vi "FPGAController_v3.vi"() -> ()   [LabVIEW 2013]
uses:
  <vilib>/rvi/interface/nirviOpenFPGA/nirviOpenFPGA.xnode
  <vilib>/rvi/interface/nirviMethod/nirviMethod.xnode
  <vilib>/rvi/interface/nirviReadWriteControl/nirviReadWriteControl.xnode
  <vilib>/rvi/interface/nirviCloseFPGA/nirviCloseFPGA.xnode
  ver1(FPGA)_7_8_2013.vi
  <vilib>/addons/database/NI_Database_API.lvlib
  <vilib>/addons/database/Recordset.llb/Rec Fetch Recordset Data (R).vi
  <vilib>/addons/database/Connection.llb/Conn Execute.vi
  <vilib>/addons/database/_DB Variant To Data/Database Variant To Data.xnode
  <vilib>/addons/database/Recordset.llb/Rec Destroy - Connection.vi
  <vilib>/Utility/miscctls.llb/LVPointTypeDef.ctl
  FPGA Bitfiles/correlationwithf_FPGATarget_ver1(FPGA)214201_RJg2enFNf9w.lvbitx
  <userlib>/_OpenG.lib/comparison/comparison.llb/Boolean Changed__ogtk.vi
  <vilib>/rvi/errors/niLvFpgaMergeErrorWithErrorCode.vi
panel:
  out "Rearm Trigger":bool
  in  "Rearm Trigger":bool
  in  "One Shot Mode":bool
  out "Last Update:":timestamp
  out "Updating FPGA":bool
  out "Sensitivity":dbl
  out "error out":errorcluster
  out "Low Mass Limit":fxp<+,31,17>
  out "High Mass Limit":fxp<+,31,17>
  out "stopping":bool
  in  "Auto Threshold":bool
  out "Peletron (MV)":dbl=2.0
  out "High Mass (kg)":dbl=inf
  out "Low Mass (kg)":dbl
  out "High Charge Limit":i16
  out "Low Charge Limit":i16
  out "High velocity count":i32=210
  out "Low velocity count":i32=21000
  in  "stop":bool
  in  "Peak-Threshold Factor":dbl=3.0
  out "Low Charge Limit (fC)":dbl
  out "High Charge Limit (fC)":dbl=100.0
  out "High Velocity":dbl=100000.0
  out "Low Velocity":dbl=1000.0
  out "Filter 7 Peak":i32=7483
  out "Filter 6 Peak":i32=9863
  out "Filter 5 Peak":i32=13910
  out "Filter 4 Peak":i32=18191
  out "Filter 3 Peak":i32=46254
  out "Filter 2 Peak":i32=120664
  out "Filter 1 Peak":i32=295996
  in  "Filter7 Threshold":i32=-21165
  in  "Filter6 Threshold":i32=-29358
  in  "Filter5 Threshold":i32=-41730
  in  "Filter4 Threshold":i32=-54306
  in  "Filter3 Threshold":i32=-138762
  in  "Filter2 Threshold":i32=-361992
  in  "Filter1 Threshold":i32=-887988
  in  "Zero Peak Values":bool
  in  "Assign Threshold":bool
  in  "Run Mode":bool
  # "Settings"
  # "Dubugging"
  # "Independent Variable"
  # "Low Vel."
  # "High Vel."
  # "Low Q (fC)"
  # "High Q (fC)"
  # "Plate Control While Loop Counter"
  # "Low Mass (kg)"
  # "High Mass (kg)"
  # "Sens. (V/pC)"
  # "Peletron (MV)"
  # "Current Value of Running Average"
  # "Peak Threshold Factor"
  # "Peak Values"
  # "Peak 1"
  # "Peak 2"
  # "Peak 3"
  # "Peak 4"
  # "Peak 5"
  # "Peak 6"
  # "Peak 7"
  # "Thresholds"
  # "Threshold 1"
  # "Threshold 2"
  # "Threshold 3"
  # "Threshold 4"
  # "Threshold 5"
  # "Threshold 6"
  # "Threshold 7"
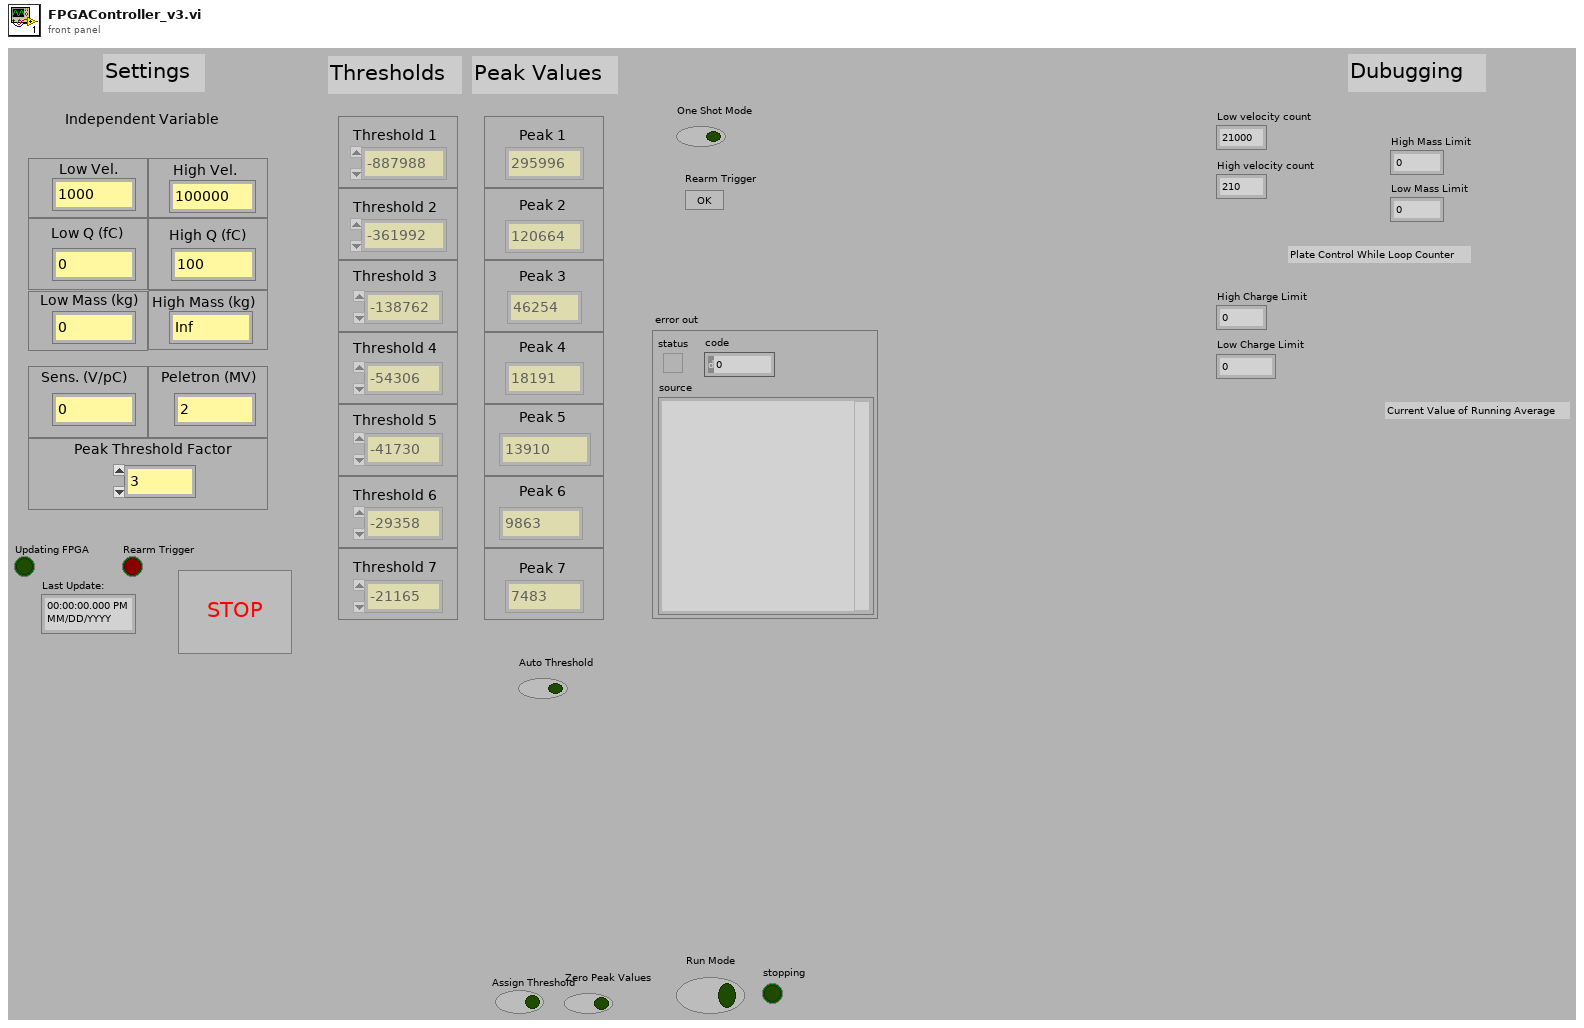
[diagram p1: front panel]
types:
  T1 = typedef "LVPointTypeDef.ctl" = cluster{"Horizontal":i16, "Vertical":i16}
  T2 = enum8{"Enabled", "Disabled", "Disabled and Grayed Out"}
  T3 = typedef "NI_Database_API.lvlib/Conn ObjectReference.ctl" = refnum<k1>
  T4 = cluster{"Filter 1 Peak":i32, "Filter 2 Peak":i32, "Filter 3 Peak":i32, "Filter 4 Peak":i32, "Filter 5 Peak":i32, "Filter 6 Peak":i32, "Filter 7 Peak":i32}
  T5 = typedef "NI_Database_API.lvlib/Rec ObjectReference.ctl" = refnum<k1>
  T6 = cluster{"Numeric":dbl, "Numeric":dbl, "Numeric":dbl, "Numeric":dbl, "Numeric":dbl, "Numeric":dbl, dbl, dbl, "Value":dbl}
  T7 = cluster{"Low Velocity Count":i32, "High Velocity Count":i32, "Low Charge Limit (ADC ticks)":i16, "High Charge Limit (ADC ticks)":i16, "Low Mass (ADC*cycle^2)":i64, "High Mass (ADC*cycle^2)":i64, "Mult":fxp<+,16,7>, "Mult Use?":bool}
  T8 = cluster{"Filter 1 Detector 3 Correlation":void, "Filter 2 Detector 3 Correlation":void, "Filter 3 Detector 3 Correlation":void, "Filter 4 Detector 3 Correlation":void, "Filter 5 Detector 3 Correlation":void, "Filter 6 Detector 3 Correlation":void, "Filter 7 Detector 3 Correlation":void}
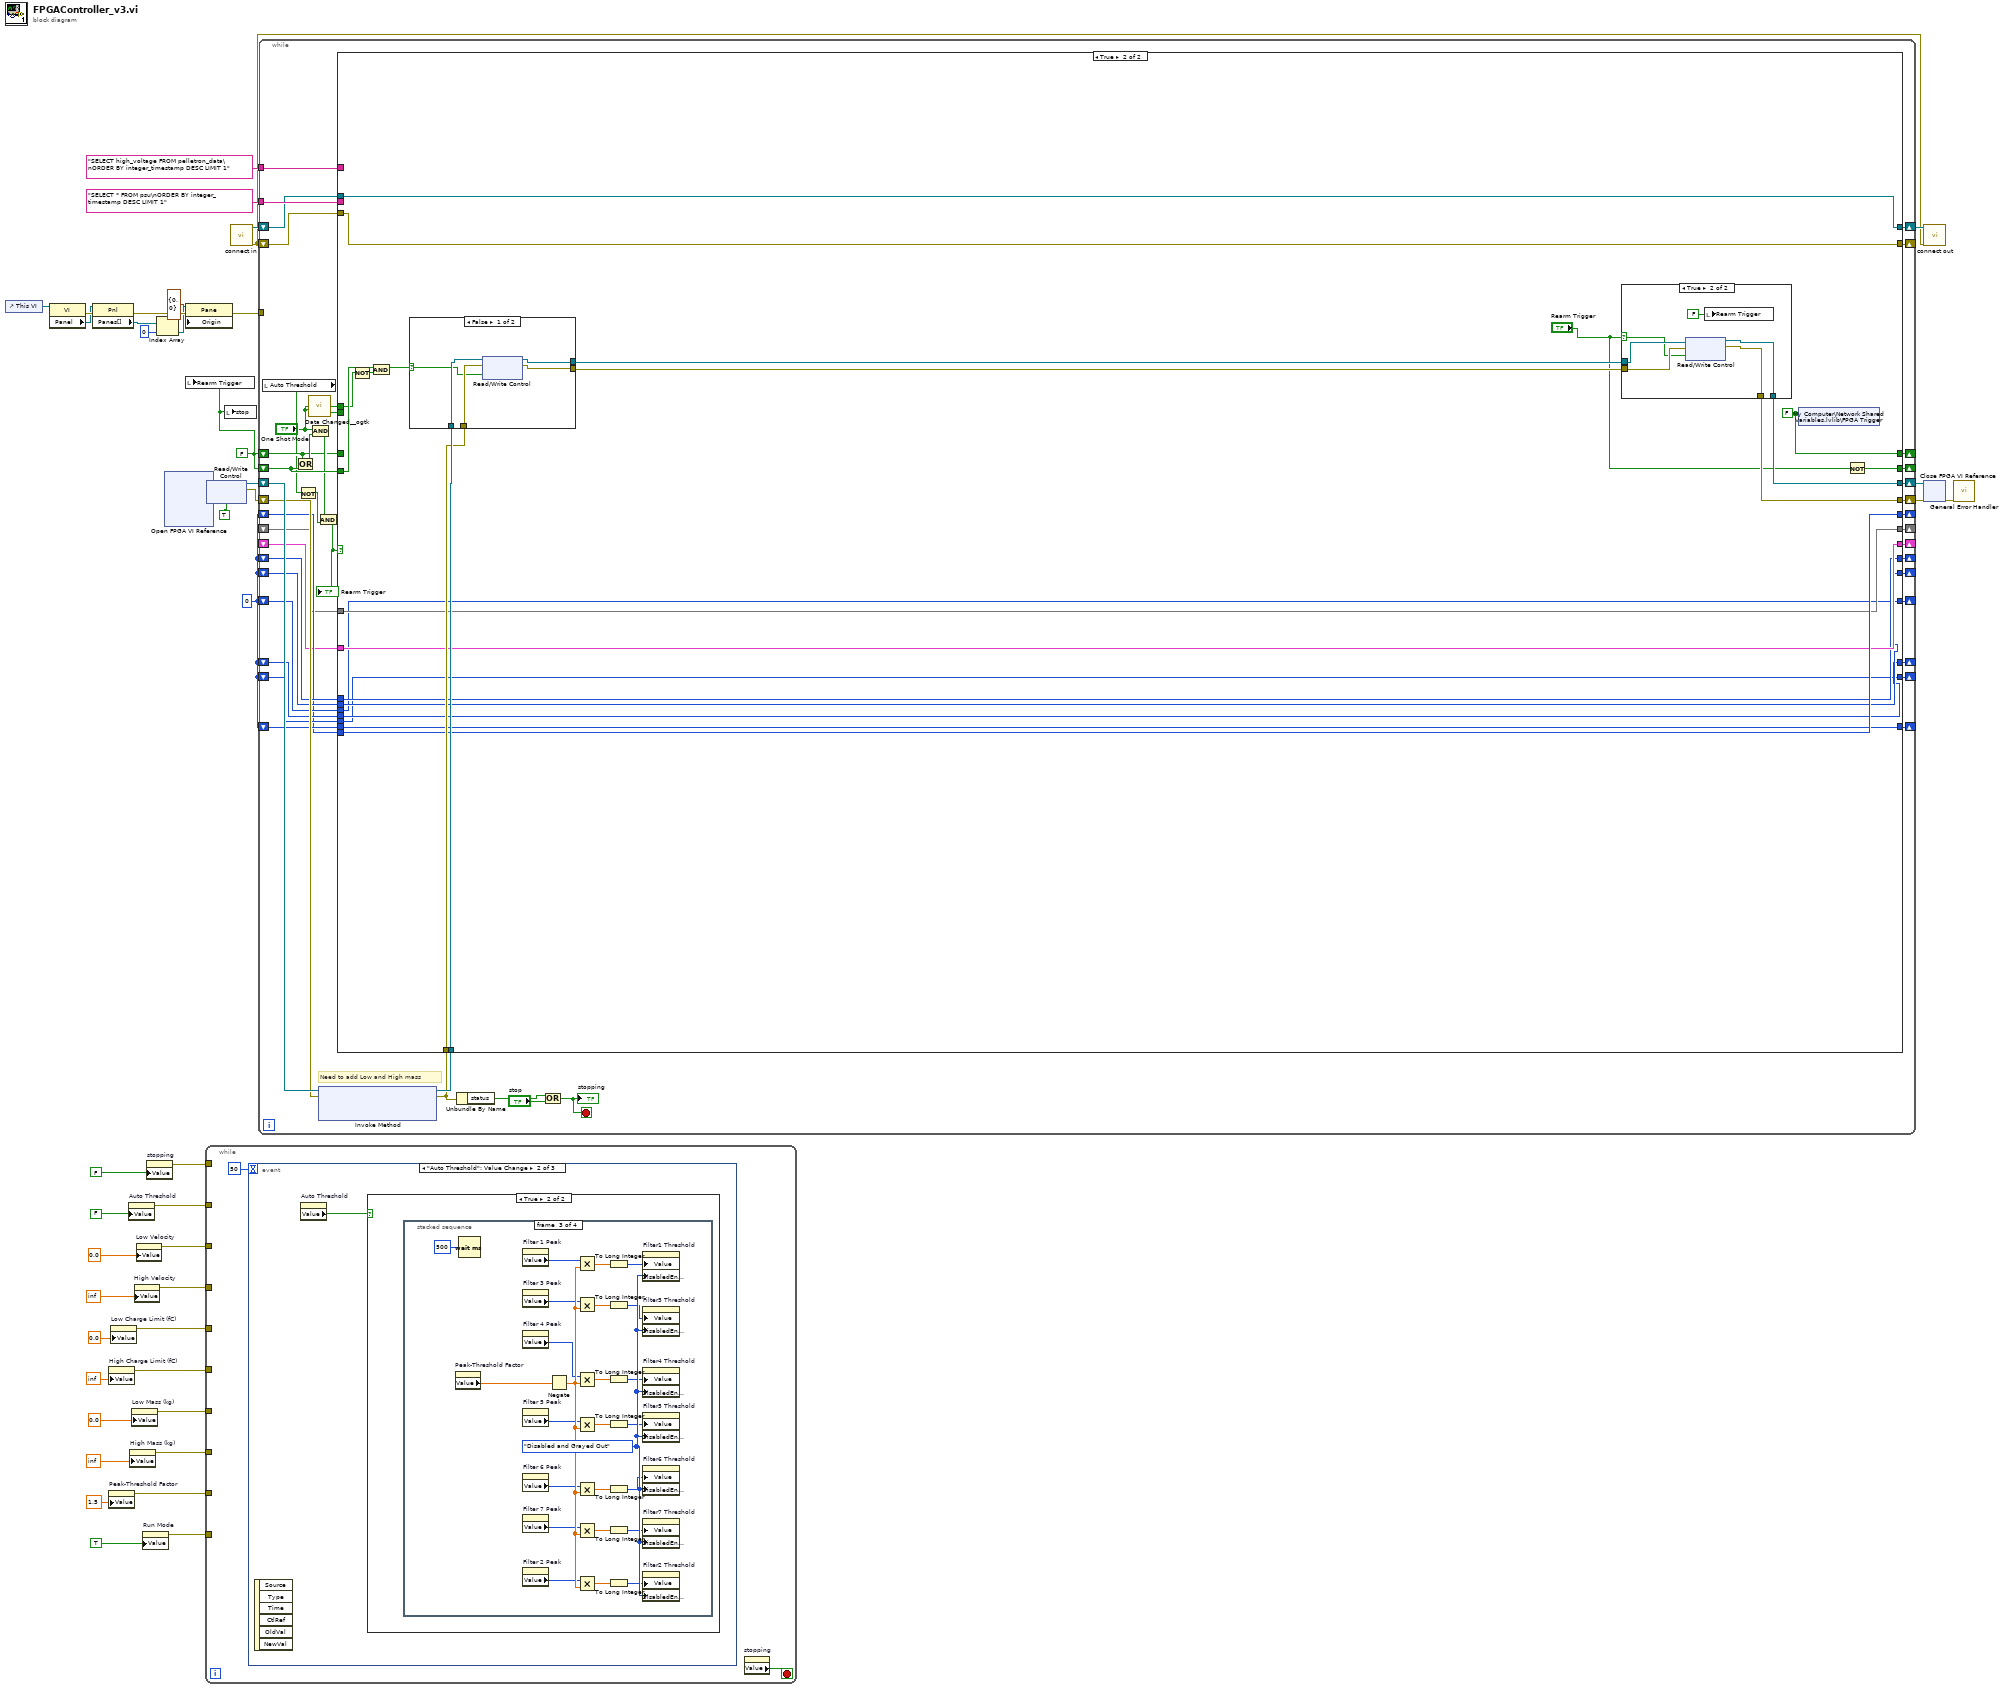
[diagram p0: block diagram]
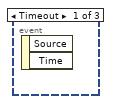
[diagram p2: hidden frame]
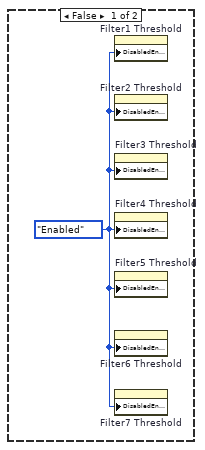
[diagram p3: hidden frame]
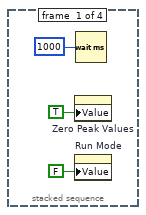
[diagram p4: hidden frame]
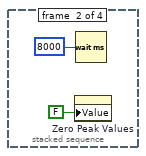
[diagram p5: hidden frame]
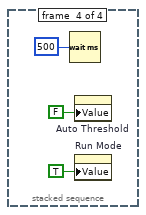
[diagram p6: hidden frame]
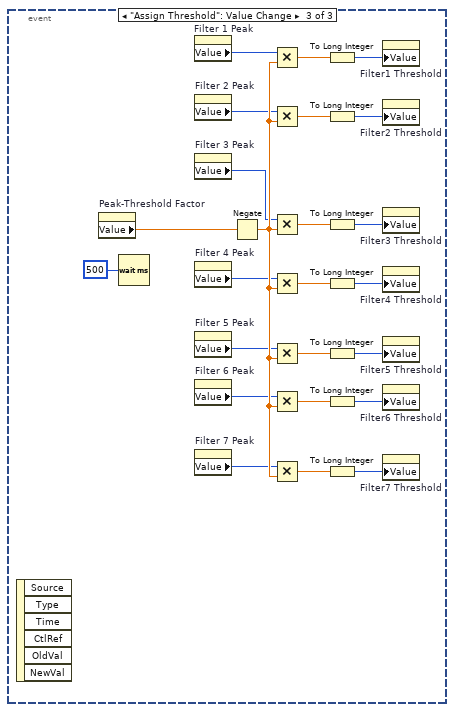
[diagram p7: hidden frame]
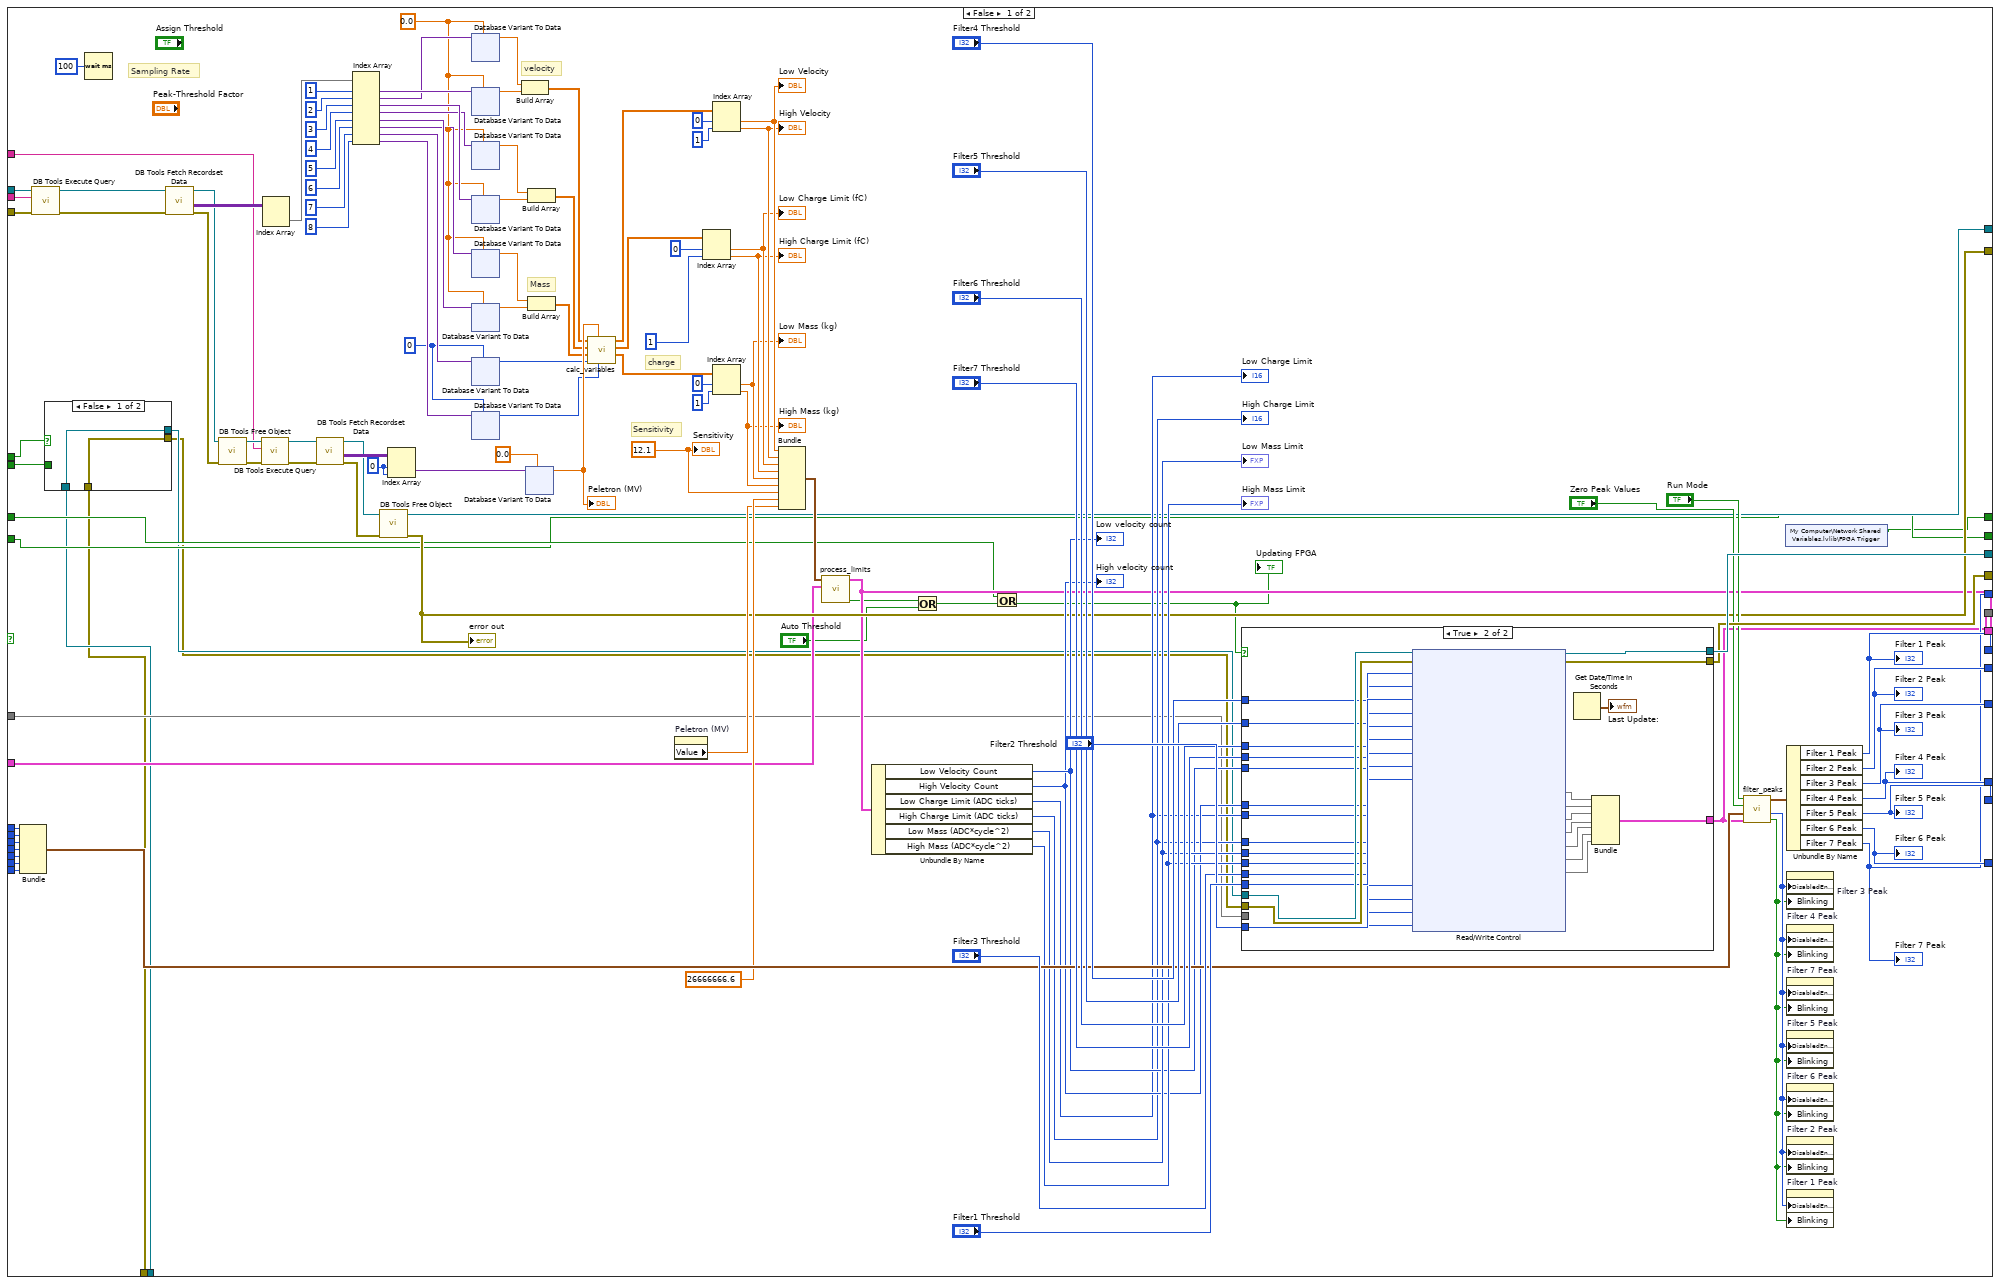
[diagram p8: hidden frame]
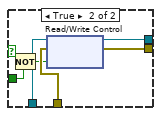
[diagram p9: hidden frame]
diagram:
  w6 = FALSE
  w43 = 0
  n1 = control-ref of="This VI"() -> (w15:refnum<vi>)
  n2 = property class="VI"(reference=w15) -> (error out=w14:errorcluster, "Panel"=w13:refnum<vi>)  [unwired: 1 in, 1 out]
  n3 = property class="Pnl"(reference=w13, error in=w14) -> (error out=w12:errorcluster, "Panes[]"=w11:refnum<vi>[])  [unwired: 1 out]
  n4 = property on="High Charge Limit (fC)" class="DigNum (strict)"("Value"=inf ("High Charge Limit (fC)")) -> (error out=w30:errorcluster)  [unwired: 2 in, 1 out]
  n5 = property on="Peak-Threshold Factor" class="DigNum (strict)"("Value"=1.5 ("Peak-Threshold Factor")) -> (error out=w24:errorcluster)  [unwired: 2 in, 1 out]
  n6 = property on="Low Charge Limit (fC)" class="DigNum (strict)"("Value"=0.0 ("Low Charge Limit (fC)")) -> (error out=w32:errorcluster)  [unwired: 2 in, 1 out]
  n7 = property on="Auto Threshold" class="Bool (strict)"("Value"=FALSE ("Auto Threshold")) -> (error out=w38:errorcluster)  [unwired: 2 in, 1 out]
  n8 = property on="High Mass (kg)" class="DigNum (strict)"("Value"=inf ("High Mass (kg)")) -> (error out=w26:errorcluster)  [unwired: 2 in, 1 out]
  n9 = property on="Low Mass (kg)" class="DigNum (strict)"("Value"=0.0 ("Low Mass (kg)")) -> (error out=w28:errorcluster)  [unwired: 2 in, 1 out]
  n10 = property on="High Velocity" class="DigNum (strict)"("Value"=inf ("High Velocity")) -> (error out=w34:errorcluster)  [unwired: 2 in, 1 out]
  n11 = property on="Low Velocity" class="DigNum (strict)"("Value"=0.0 ("Low Velocity")) -> (error out=w36:errorcluster)  [unwired: 2 in, 1 out]
  n12 = property on="Run Mode" class="Bool (strict)"("Value"=TRUE ("Run Mode")) -> (error out=w22:errorcluster)  [unwired: 2 in, 1 out]
  n13 = property on="stopping" class="Bool (strict)"("Value"=FALSE ("stopping")) -> (error out=w40:errorcluster)  [unwired: 2 in, 1 out]
  n14 = Index Array(array=w11, index=0) -> (element=w9:refnum<vi>)
  n15 = xnode "Open FPGA VI Reference"() -> ("FPGA VI Reference Out"=w5:refnum<k20>, "error out"=w4:errorcluster)  [unwired: 2 in]
  n16 = property class="Pane"(reference=w9, error in=w12, "Origin"=T1 {"Horizontal"=0, "Vertical"=0}) -> (error out=w7:errorcluster)  [unwired: 1 out]
  n17 = local write "Rearm Trigger"(w6) -> ()
  n18 = while {
    tunnel: w40 -> [_]
    tunnel: w38 -> [_]
    tunnel: w36 -> [_]
    tunnel: w34 -> [_]
    tunnel: w32 -> [_]
    tunnel: w30 -> [_]
    tunnel: w28 -> [_]
    tunnel: w26 -> [_]
    tunnel: w24 -> [_]
    tunnel: w22 -> [_]
    stop <- w46 stop-if-true
    n19 = event shown="[1] \"Auto Threshold\": Value Change" {
      selector: _ -> [_ _ _]
      dyn-events: _ -> [_ _ _]
      timeout: 50 -> [_ _ _]
      event Timeout {
        n20 = event-data() -> ()  [unwired: 1 in, 2 out]
      }
      event "Auto Threshold": Value Change {
        n21 = event-data() -> ()  [unwired: 1 in, 6 out]
        n22 = property on="Auto Threshold" class="Bool (strict)"() -> ("Value"=w47:bool)  [unwired: 2 in, 2 out]
        n23 = case shown="True" w47 {
          frame False {
            w48 = T2."Enabled" ("Disabled")
            n24 = property on="Filter1 Threshold" class="DigNum (strict)"("DisabledEnum"=w48) -> ()  [unwired: 2 in, 2 out]
            n25 = property on="Filter2 Threshold" class="DigNum (strict)"("DisabledEnum"=w48) -> ()  [unwired: 2 in, 2 out]
            n26 = property on="Filter3 Threshold" class="DigNum (strict)"("DisabledEnum"=w48) -> ()  [unwired: 2 in, 2 out]
            n27 = property on="Filter4 Threshold" class="DigNum (strict)"("DisabledEnum"=w48) -> ()  [unwired: 2 in, 2 out]
            n28 = property on="Filter5 Threshold" class="DigNum (strict)"("DisabledEnum"=w48) -> ()  [unwired: 2 in, 2 out]
            n29 = property on="Filter6 Threshold" class="DigNum (strict)"("DisabledEnum"=w48) -> ()  [unwired: 2 in, 2 out]
            n30 = property on="Filter7 Threshold" class="DigNum (strict)"("DisabledEnum"=w48) -> ()  [unwired: 2 in, 2 out]
          }
          frame True {
            n31 = stacked-sequence {
              frame #0 {
                n32 = property on="Zero Peak Values" class="Bool (strict)"("Value"=TRUE ("Zero Peak Values")) -> ()  [unwired: 2 in, 2 out]
                n33 = property on="Run Mode" class="Bool (strict)"("Value"=FALSE ("Run Mode")) -> ()  [unwired: 2 in, 2 out]
                n34 = Wait (ms)(milliseconds to wait=u32 1000) -> ()  [unwired: 1 out]
              }
              frame #1 {
                n35 = property on="Zero Peak Values" class="Bool (strict)"("Value"=FALSE ("Zero Peak Values")) -> ()  [unwired: 2 in, 2 out]
                n36 = Wait (ms)(milliseconds to wait=u32 8000) -> ()  [unwired: 1 out]
              }
              frame #2 {
                w78 = T2."Disabled and Grayed Out" ("Disabled")
                n37 = property on="Peak-Threshold Factor" class="DigNum (strict)"() -> ("Value"=w63:dbl)  [unwired: 2 in, 2 out]
                n38 = Wait (ms)(milliseconds to wait=u32 500) -> ()  [unwired: 1 out]
                n39 = property on="Filter 1 Peak" class="DigNum (strict)"() -> ("Value"=w61:i32)  [unwired: 2 in, 2 out]
                n40 = property on="Filter 3 Peak" class="DigNum (strict)"() -> ("Value"=w59:i32)  [unwired: 2 in, 2 out]
                n41 = property on="Filter 4 Peak" class="DigNum (strict)"() -> ("Value"=w58:i32)  [unwired: 2 in, 2 out]
                n42 = property on="Filter 5 Peak" class="DigNum (strict)"() -> ("Value"=w57:i32)  [unwired: 2 in, 2 out]
                n43 = property on="Filter 6 Peak" class="DigNum (strict)"() -> ("Value"=w56:i32)  [unwired: 2 in, 2 out]
                n44 = property on="Filter 7 Peak" class="DigNum (strict)"() -> ("Value"=w55:i32)  [unwired: 2 in, 2 out]
                n45 = property on="Filter 2 Peak" class="DigNum (strict)"() -> ("Value"=w60:i32)  [unwired: 2 in, 2 out]
                n46 = Negate(x=w63) -> (-x=w62:dbl)
                n47 = Multiply(x=w61, y=w62) -> (x*y=w77:dbl)
                n48 = Multiply(x=w59, y=w62) -> (x*y=w73:dbl)
                n49 = Multiply(x=w58, y=w62) -> (x*y=w71:dbl)
                n50 = Multiply(x=w57, y=w62) -> (x*y=w69:dbl)
                n51 = Multiply(x=w56, y=w62) -> (x*y=w67:dbl)
                n52 = Multiply(x=w55, y=w62) -> (x*y=w65:dbl)
                n53 = Multiply(x=w60, y=w62) -> (x*y=w75:dbl)
                n54 = To Long Integer(number=w77) -> (32bit integer=w76:i32)
                n55 = To Long Integer(number=w73) -> (32bit integer=w72:i32)
                n56 = To Long Integer(number=w71) -> (32bit integer=w70:i32)
                n57 = To Long Integer(number=w69) -> (32bit integer=w68:i32)
                n58 = To Long Integer(number=w67) -> (32bit integer=w66:i32)
                n59 = To Long Integer(number=w65) -> (32bit integer=w64:i32)
                n60 = To Long Integer(number=w75) -> (32bit integer=w74:i32)
                n61 = property on="Filter1 Threshold" class="DigNum (strict)"("Value"=w76, "DisabledEnum"=w78) -> ()  [unwired: 2 in, 2 out]
                n62 = property on="Filter3 Threshold" class="DigNum (strict)"("Value"=w72, "DisabledEnum"=w78) -> ()  [unwired: 2 in, 2 out]
                n63 = property on="Filter4 Threshold" class="DigNum (strict)"("Value"=w70, "DisabledEnum"=w78) -> ()  [unwired: 2 in, 2 out]
                n64 = property on="Filter5 Threshold" class="DigNum (strict)"("Value"=w68, "DisabledEnum"=w78) -> ()  [unwired: 2 in, 2 out]
                n65 = property on="Filter6 Threshold" class="DigNum (strict)"("Value"=w66, "DisabledEnum"=w78) -> ()  [unwired: 2 in, 2 out]
                n66 = property on="Filter7 Threshold" class="DigNum (strict)"("Value"=w64, "DisabledEnum"=w78) -> ()  [unwired: 2 in, 2 out]
                n67 = property on="Filter2 Threshold" class="DigNum (strict)"("Value"=w74, "DisabledEnum"=w78) -> ()  [unwired: 2 in, 2 out]
              }
              frame #3 {
                n68 = Wait (ms)(milliseconds to wait=u32 500) -> ()  [unwired: 1 out]
                n69 = property on="Auto Threshold" class="Bool (strict)"("Value"=FALSE ("Auto Threshold")) -> ()  [unwired: 2 in, 2 out]
                n70 = property on="Run Mode" class="Bool (strict)"("Value"=TRUE ("Run Mode")) -> ()  [unwired: 2 in, 2 out]
              }
            }
          }
        }
      }
      event "Assign Threshold": Value Change {
        n71 = event-data() -> ()  [unwired: 1 in, 6 out]
        n72 = property on="Peak-Threshold Factor" class="DigNum (strict)"() -> ("Value"=w96:dbl)  [unwired: 2 in, 2 out]
        n73 = Wait (ms)(milliseconds to wait=u32 500) -> ()  [unwired: 1 out]
        n74 = property on="Filter 1 Peak" class="DigNum (strict)"() -> ("Value"=w95:i32)  [unwired: 2 in, 2 out]
        n75 = property on="Filter 2 Peak" class="DigNum (strict)"() -> ("Value"=w94:i32)  [unwired: 2 in, 2 out]
        n76 = property on="Filter 3 Peak" class="DigNum (strict)"() -> ("Value"=w93:i32)  [unwired: 2 in, 2 out]
        n77 = property on="Filter 4 Peak" class="DigNum (strict)"() -> ("Value"=w92:i32)  [unwired: 2 in, 2 out]
        n78 = property on="Filter 5 Peak" class="DigNum (strict)"() -> ("Value"=w91:i32)  [unwired: 2 in, 2 out]
        n79 = property on="Filter 6 Peak" class="DigNum (strict)"() -> ("Value"=w90:i32)  [unwired: 2 in, 2 out]
        n80 = property on="Filter 7 Peak" class="DigNum (strict)"() -> ("Value"=w89:i32)  [unwired: 2 in, 2 out]
        n81 = Negate(x=w96) -> (-x=w98:dbl)
        n82 = Multiply(x=w95, y=w98) -> (x*y=w105:dbl)
        n83 = Multiply(x=w94, y=w98) -> (x*y=w103:dbl)
        n84 = Multiply(x=w93, y=w98) -> (x*y=w102:dbl)
        n85 = Multiply(x=w92, y=w98) -> (x*y=w101:dbl)
        n86 = Multiply(x=w91, y=w98) -> (x*y=w100:dbl)
        n87 = Multiply(x=w90, y=w98) -> (x*y=w99:dbl)
        n88 = Multiply(x=w89, y=w98) -> (x*y=w104:dbl)
        n89 = To Long Integer(number=w105) -> (32bit integer=w88:i32)
        n90 = To Long Integer(number=w103) -> (32bit integer=w87:i32)
        n91 = To Long Integer(number=w102) -> (32bit integer=w86:i32)
        n92 = To Long Integer(number=w101) -> (32bit integer=w85:i32)
        n93 = To Long Integer(number=w100) -> (32bit integer=w84:i32)
        n94 = To Long Integer(number=w99) -> (32bit integer=w83:i32)
        n95 = To Long Integer(number=w104) -> (32bit integer=w82:i32)
        n96 = property on="Filter1 Threshold" class="DigNum (strict)"("Value"=w88) -> ()  [unwired: 2 in, 2 out]
        n97 = property on="Filter2 Threshold" class="DigNum (strict)"("Value"=w87) -> ()  [unwired: 2 in, 2 out]
        n98 = property on="Filter3 Threshold" class="DigNum (strict)"("Value"=w86) -> ()  [unwired: 2 in, 2 out]
        n99 = property on="Filter4 Threshold" class="DigNum (strict)"("Value"=w85) -> ()  [unwired: 2 in, 2 out]
        n100 = property on="Filter5 Threshold" class="DigNum (strict)"("Value"=w84) -> ()  [unwired: 2 in, 2 out]
        n101 = property on="Filter6 Threshold" class="DigNum (strict)"("Value"=w83) -> ()  [unwired: 2 in, 2 out]
        n102 = property on="Filter7 Threshold" class="DigNum (strict)"("Value"=w82) -> ()  [unwired: 2 in, 2 out]
      }
    }
    n103 = property on="stopping" class="Bool (strict)"() -> ("Value"=w46:bool)  [unwired: 2 in, 2 out]
  }
  n104 = xnode "Read/Write Control"("FPGA VI Reference In"=w5, "error in"=w4, "Output"=TRUE) -> ("FPGA VI Reference Out"=w2:refnum<k20>, "error out"=w3:errorcluster)
  n105 = local write "stop"(w6) -> ()
  n106 = call "connect in.vi"() -> ("error out"=w16:errorcluster, "Database Connection"=w17:T3)  [unwired: 7 in, 1 out]
  n107 = while {
    shift-right: [w143] -> w42
    shift-left: w2 -> [w149]
    shift-right: [w142] -> w41
    shift-left: w3 -> [w148]
    shift-right: [w138] -> _
    shift-left: w43 -> [w131]
    shift-right: [w137] -> _
    shift-left: w43 -> [w130]
    shift-right: [w136] -> _
    shift-left: w43 -> [w129]
    shift-right: [w135] -> _
    shift-left: w43 -> [w128]
    shift-right: [w134] -> _
    shift-left: w43 -> [w127]
    shift-right: [w140] -> _
    shift-left: w43 -> [w133]
    shift-right: [w139] -> _
    shift-left: w43 -> [w132]
    tunnel: "SELECT * FROM psu\nORDER BY integer_timestamp DESC LIMIT 1" ("SQL query") -> [w126]
    tunnel: "SELECT high_voltage FROM pelletron_data\nORDER BY integer_timestamp DESC LIMIT 1" ("SQL query") -> [w125]
    shift-right: [w121] -> w18
    shift-left: w17 -> [w124]
    shift-right: [w122] -> _
    shift-left: w16 -> [w123]
    shift-right: [w120] -> _
    shift-left: _ -> [w119]
    shift-right: [w117] -> _
    shift-left: _ -> [w118]
    tunnel: w7 -> [_]
    shift-right: [w116] -> _
    shift-left: w6 -> [w111]
    shift-right: [w114] -> _
    shift-left: w6 -> [w115]
    stop <- w141 stop-if-true
    # "Need to add Low and High mass"
    n108 = local read "Auto Threshold"() -> (w109:bool)
    n109 = Or(x=w111, y=w115) -> (x .or. y?=w112:bool)
    n110 = Not(x=w109) -> (.not. x?=w108:bool)
    n111 = call-poly <userlib>:"Data Changed__ogtk.vi"("Boolean"="One Shot Mode") -> ("Changed"=w107:bool)
    n112 = And(x="One Shot Mode", y=w112) -> (x .and. y?=w113:bool)
    n113 = And(x=w113, y=w108) -> (x .and. y?=w110:bool)
    "Rearm Trigger" <- w110
    n114 = xnode "Invoke Method"("FPGA VI Reference In"=w149, "error in"=w148) -> ("FPGA VI Reference Out"=w145:refnum<k20>, "error out"=w144:errorcluster)  [unwired: 1 out]
    n115 = case shown="True" w110 {
      tunnel: w145 -> [w153 w619]
      tunnel: w144 -> [w151 w618]
      tunnel: [w273 w617] -> w143
      tunnel: [w272 w614] -> w142
      tunnel: [w261 w608] -> w140
      tunnel: [w260 w607] -> w139
      tunnel: [w259 w606] -> w138
      tunnel: [w258 w605] -> w137
      tunnel: [w257 w604] -> w136
      tunnel: [w256 w603] -> w135
      tunnel: [w255 w611] -> w134
      tunnel: w133 -> [w254 w608]
      tunnel: w132 -> [w253 w607]
      tunnel: w131 -> [w252 w606]
      tunnel: w130 -> [w251 w605]
      tunnel: w129 -> [w250 w604]
      tunnel: w128 -> [w249 w603]
      tunnel: w127 -> [w248 w611]
      tunnel: w126 -> [w236 _]
      tunnel: w125 -> [w209 _]
      tunnel: w124 -> [w174 w622]
      tunnel: w123 -> [w173 w621]
      tunnel: [w170 w621] -> w122
      tunnel: [w169 w622] -> w121
      tunnel: [w167 w609] -> w120
      tunnel: w119 -> [w166 w609]
      tunnel: w118 -> [w162 w610]
      tunnel: [w161 w610] -> w117
      tunnel: w111 -> [w158 _]
      tunnel: [w156 w602] -> w116
      tunnel: w115 -> [w157 w620]
      tunnel: [w157 w612] -> w114
      tunnel: w107 -> [w155 w600]
      tunnel: "One Shot Mode" -> [w154 _]
      frame False {
        w205 = 0 ("index (row)")
        w214 = i8 0
        w215 = 0.0
        w168 = 12.1
        # "Mass"
        # "charge"
        # "velocity"
        # "Sensitivity"
        # "Sampling Rate"
        n116 = Bundle("Filter 1 Peak"=w254, "Filter 2 Peak"=w253, "Filter 3 Peak"=w252, "Filter 4 Peak"=w251, "Filter 5 Peak"=w250, "Filter 6 Peak"=w249, "Filter 7 Peak"=w248) -> (w247:T4)  [unwired: 1 in]
        n117 = call-poly <vilib>:"DB Tools Execute Query.vi"("error in (no error)"=w173, "SQL query"=w236, "connection reference"=w174) -> ("error out"=w234:errorcluster, "recordset reference"=w235:T5)  [unwired: 5 in]
        n118 = case shown="False" w155 {
          tunnel: w154 -> [_ w279]
          tunnel: w153 -> [w275 w281]
          tunnel: w151 -> [w274 w280]
          tunnel: [w274 w277] -> w150
          tunnel: [w275 w276] -> w152
          frame False {
          }
          frame True {
            n119 = Not(x=w279) -> (.not. x?=w278:bool)
            n120 = xnode "Read/Write Control"("FPGA VI Reference In"=w281, "error in"=w280, "Output"=w278) -> ("FPGA VI Reference Out"=w276:refnum<k20>, "error out"=w277:errorcluster)
          }
        }
        n121 = Wait (ms)(milliseconds to wait=u32 100) -> ()  [unwired: 1 out]
        n122 = call-poly <vilib>:"DB Tools Fetch Recordset Data.vi"("error in (no error)"=w234, "recordset reference"=w235) -> ("error out"=w212:errorcluster, "recordset data"=w225:variant[][], "recordset reference out"=w213:T5)  [unwired: 3 in]
        n123 = call-poly <vilib>:"DB Tools Free Object.vi"("error in (no error)"=w212, "recordset reference"=w213) -> ("error out"=w210:errorcluster, "connection reference"=w211:T3)  [unwired: 8 in]
        n124 = call-poly <vilib>:"DB Tools Execute Query.vi"("error in (no error)"=w210, "SQL query"=w209, "connection reference"=w211) -> ("error out"=w207:errorcluster, "recordset reference"=w208:T5)  [unwired: 5 in]
        n125 = Index Array(array=w225) -> (element=w224:variant[])  [unwired: 2 in]
        n126 = call-poly <vilib>:"DB Tools Fetch Recordset Data.vi"("error in (no error)"=w207, "recordset reference"=w208) -> ("error out"=w171:errorcluster, "recordset data"=w206:variant[][], "recordset reference out"=w172:T5)  [unwired: 3 in]
        n127 = Index Array(array=w224, index #1=1 ("index"), index #2=2 ("index"), index #3=3 ("index"), index #4=4 ("index"), index #5=5 ("index"), index #6=6 ("index"), index #7=7 ("index"), index #8=8 ("index")) -> (element #1=w223:variant, element #2=w222:variant, element #3=w221:variant, element #4=w220:variant, element #5=w219:variant, element #6=w218:variant, element #7=w217:variant, element #8=w216:variant)
        n128 = call-poly <vilib>:"DB Tools Free Object.vi"("error in (no error)"=w171, "recordset reference"=w172) -> ("error out"=w170:errorcluster, "connection reference"=w169:T3)  [unwired: 8 in]
        "error out" <- w170
        n129 = Index Array(array=w206, index (row)=w205, index (col)=w205) -> (element=w204:variant)
        n130 = xnode "Database Variant To Data"("database variant"=w222, "type"=w215) -> ("data"=w201:dbl)  [unwired: 1 in, 1 out]
        n131 = xnode "Database Variant To Data"("database variant"=w223, "type"=w215) -> ("data"=w200:dbl)  [unwired: 1 in, 1 out]
        n132 = xnode "Database Variant To Data"("database variant"=w220, "type"=w215) -> ("data"=w199:dbl)  [unwired: 1 in, 1 out]
        n133 = xnode "Database Variant To Data"("database variant"=w221, "type"=w215) -> ("data"=w198:dbl)  [unwired: 1 in, 1 out]
        n134 = xnode "Database Variant To Data"("database variant"=w218, "type"=w215) -> ("data"=w197:dbl)  [unwired: 1 in, 1 out]
        n135 = xnode "Database Variant To Data"("database variant"=w219, "type"=w215) -> ("data"=w196:dbl)  [unwired: 1 in, 1 out]
        n136 = xnode "Database Variant To Data"("database variant"=w217, "type"=w214) -> ("data"=w191:i8)  [unwired: 1 in, 1 out]
        n137 = xnode "Database Variant To Data"("database variant"=w216, "type"=w214) -> ("data"=w190:i8)  [unwired: 1 in, 1 out]
        n138 = Build Array(w201, w200) -> (w194:dbl[])
        n139 = xnode "Database Variant To Data"("database variant"=w204, "type"=0.0) -> ("data"=w195:dbl)  [unwired: 1 in, 1 out]
        "Peletron (MV)" <- w195
        n140 = Build Array(w199, w198) -> (w193:dbl[])
        n141 = Build Array(w197, w196) -> (w192:dbl[])
        n142 = call "calc_variables.vi"("var2"=w190, "Peletron"=w195, "var1"=w191, "Mass"=w192, "Charge"=w193, "Velocity"=w194) -> ("Mass out"=w183:dbl[], "Charge out"=w186:dbl[], "Velocity out"=w189:dbl[])  [unwired: 3 in]
        n143 = property on="Peletron (MV)" class="DigNum (strict)"() -> ("Value"=w202:dbl)  [unwired: 2 in, 2 out]
        n144 = Index Array(array=w186, index #1=0 ("index"), index #2=1 ("index")) -> (element #1=w178:dbl, element #2=w177:dbl)
        "High Charge Limit (fC)" <- w177
        "Low Charge Limit (fC)" <- w178
        n145 = Index Array(array=w189, index #1=0 ("index"), index #2=1 ("index")) -> (element #1=w180:dbl, element #2=w179:dbl)
        "High Velocity" <- w179
        "Low Velocity" <- w180
        n146 = Index Array(array=w183, index #1=0 ("index"), index #2=1 ("index")) -> (element #1=w176:dbl, element #2=w175:dbl)
        "Low Mass (kg)" <- w176
        "High Mass (kg)" <- w175
        n147 = Bundle("Numeric"=w180, "Numeric"=w179, "Numeric"=w178, "Numeric"=w177, "Numeric"=w176, "Numeric"=w175, w168, 26666666.6, "Value"=w202) -> (w246:T6)  [unwired: 1 in]
        n148 = call "process_limits.vi"("old output cluster"=w166, "Input cluster"=w246) -> ("Update FPGA"=w163:bool, "output cluster"=w167:T7)  [unwired: 8 in]
        n149 = Unbundle By Name(w167) -> ("Low Velocity Count"=w242:i32, "High Velocity Count"=w241:i32, "Low Charge Limit (ADC ticks)"=w239:i16, "High Charge Limit (ADC ticks)"=w240:i16, "Low Mass (ADC*cycle^2)"=w244:i64, "High Mass (ADC*cycle^2)"=w245:i64)
        "Low velocity count" <- w242
        "High velocity count" <- w241
        "High Charge Limit" <- w240
        "Low Charge Limit" <- w239
        "High Mass Limit" <- w245
        "Low Mass Limit" <- w244
        n150 = Or(x=w163, y="Auto Threshold") -> (x .or. y?=w165:bool)
        n151 = Or(x=w158, y=w165) -> (x .or. y?=w159:bool)
        "Updating FPGA" <- w159
        n152 = case shown="True" w159 {
          tunnel: w152 -> [w283 w310]
          tunnel: w150 -> [w284 w309]
          tunnel: [w283 w308] -> w273
          tunnel: [w284 w307] -> w272
          tunnel: "Filter1 Threshold" -> [_ w306]
          tunnel: "Filter2 Threshold" -> [_ w305]
          tunnel: "Filter3 Threshold" -> [_ w304]
          tunnel: "Filter4 Threshold" -> [_ w303]
          tunnel: "Filter5 Threshold" -> [_ w302]
          tunnel: "Filter6 Threshold" -> [_ w301]
          tunnel: "Filter7 Threshold" -> [_ w300]
          tunnel: [w282 w286] -> w161
          tunnel: w245 -> [_ w292]
          tunnel: w244 -> [_ w291]
          tunnel: w242 -> [_ w290]
          tunnel: w241 -> [_ w289]
          tunnel: w240 -> [_ w288]
          tunnel: w239 -> [_ w287]
          tunnel: w162 -> [w282 _]
          frame False {
          }
          frame True {
            n153 = xnode "Read/Write Control"("FPGA VI Reference In"=w310, "error in"=w309, "Low Velocity Count"=w290, "High Velocity Count"=w289, "Filter 1 threshold"=w306, "Filter 2 threshold"=w305, "Filter 3 threshold"=w304, "Filter 4 threshold"=w303, "Filter 5 threshold"=w302, "Filter 6 threshold"=w301, "Filter 7 threshold"=w300, "High Charge Limit"=w288, "Low Charge Limit"=w287, "High Mass Limit"=w292, "Low Mass Limit"=w291) -> ("FPGA VI Reference Out"=w308:refnum<k20>, "error out"=w307:errorcluster, "Filter 1 Detector 3 Correlation"=w299, "Filter 2 Detector 3 Correlation"=w298, "Filter 3 Detector 3 Correlation"=w297, "Filter 4 Detector 3 Correlation"=w296, "Filter 5 Detector 3 Correlation"=w295, "Filter 6 Detector 3 Correlation"=w294, "Filter 7 Detector 3 Correlation"=w293)
            n154 = Get Date/Time In Seconds() -> (seconds since 1Jan1904=→"Last Update:":timestamp)
            n155 = Bundle("Filter 1 Detector 3 Correlation"=w299, "Filter 2 Detector 3 Correlation"=w298, "Filter 3 Detector 3 Correlation"=w297, "Filter 4 Detector 3 Correlation"=w296, "Filter 5 Detector 3 Correlation"=w295, "Filter 6 Detector 3 Correlation"=w294, "Filter 7 Detector 3 Correlation"=w293) -> (w286:T8)  [unwired: 1 in]
          }
        }
        n156 = call "filter_peaks.vi"("Correlation cluster"=w161, "Filter peak cluster"=w247, "Zero out"="Zero Peak Values", "Run Mode"="Run Mode") -> ("Blinking"=w238:bool, "status"=w243:T2, "Filter peak output"=w262:T4)  [unwired: 5 in]
        n157 = shared-variable "My Computer\\Network Shared Variables.lvlib\\FPGA Trigger"() -> (w156:bool)  [unwired: 1 in, 1 out]
        n158 = Unbundle By Name(w262) -> ("Filter 1 Peak"=w261:i32, "Filter 2 Peak"=w260:i32, "Filter 3 Peak"=w259:i32, "Filter 4 Peak"=w258:i32, "Filter 5 Peak"=w257:i32, "Filter 6 Peak"=w256:i32, "Filter 7 Peak"=w255:i32)
        "Filter 1 Peak" <- w261
        "Filter 2 Peak" <- w260
        "Filter 3 Peak" <- w259
        "Filter 4 Peak" <- w258
        "Filter 5 Peak" <- w257
        "Filter 6 Peak" <- w256
        "Filter 7 Peak" <- w255
        n159 = property on="Filter 3 Peak" class="DigNum (strict)"("DisabledEnum"=w243, "Blinking"=w238) -> ()  [unwired: 2 in, 2 out]
        n160 = property on="Filter 4 Peak" class="DigNum (strict)"("DisabledEnum"=w243, "Blinking"=w238) -> ()  [unwired: 2 in, 2 out]
        n161 = property on="Filter 7 Peak" class="DigNum (strict)"("DisabledEnum"=w243, "Blinking"=w238) -> ()  [unwired: 2 in, 2 out]
        n162 = property on="Filter 5 Peak" class="DigNum (strict)"("DisabledEnum"=w243, "Blinking"=w238) -> ()  [unwired: 2 in, 2 out]
        n163 = property on="Filter 6 Peak" class="DigNum (strict)"("DisabledEnum"=w243, "Blinking"=w238) -> ()  [unwired: 2 in, 2 out]
        n164 = property on="Filter 2 Peak" class="DigNum (strict)"("DisabledEnum"=w243, "Blinking"=w238) -> ()  [unwired: 2 in, 2 out]
        n165 = property on="Filter 1 Peak" class="DigNum (strict)"("DisabledEnum"=w243, "Blinking"=w238) -> ()  [unwired: 2 in, 2 out]
        "Sensitivity" <- w168
      }
      frame True {
        w602 = FALSE ("FPGA Trigger")
        n166 = Not(x=w600) -> (.not. x?=w599:bool)
        n167 = And(x=w620, y=w599) -> (x .and. y?=w601:bool)
        n168 = case shown="False" w601 {
          selector: w601 -> [w625 _]
          tunnel: w619 -> [w627 w629]
          tunnel: [w624 w629] -> w616
          tunnel: w618 -> [w626 w628]
          tunnel: [w623 w628] -> w615
          frame False {
            n169 = xnode "Read/Write Control"("FPGA VI Reference In"=w627, "error in"=w626, "Output"=w625) -> ("FPGA VI Reference Out"=w624:refnum<k20>, "error out"=w623:errorcluster)
          }
          frame True {
          }
        }
        n170 = case shown="True" "Rearm Trigger" {
          selector: "Rearm Trigger" -> [_ w632]
          tunnel: w616 -> [w631 w636]
          tunnel: [w631 w633] -> w617
          tunnel: w615 -> [w630 w635]
          tunnel: [w630 w634] -> w614
          frame False {
          }
          frame True {
            n171 = xnode "Read/Write Control"("FPGA VI Reference In"=w636, "error in"=w635, "Output"=w632) -> ("FPGA VI Reference Out"=w633:refnum<k20>, "error out"=w634:errorcluster)
            n172 = local write "Rearm Trigger"(FALSE ("Rearm Trigger")) -> ()
          }
        }
        n173 = shared-variable "My Computer\\Network Shared Variables.lvlib\\FPGA Trigger"(w602) -> ()  [unwired: 1 in, 1 out]
        n174 = Not(x="Rearm Trigger") -> (.not. x?=w612:bool)
      }
    }
    n175 = Unbundle By Name(w144) -> ("status"=w147:bool)
    n176 = Or(x=w147, y="stop") -> (x .or. y?=w141:bool)
    "stopping" <- w141
  }
  n177 = call "connect out.vi"("error in (no error)"=w16, "connection reference"=w18) -> ()  [unwired: 9 in, 1 out]
  n178 = xnode "Close FPGA VI Reference"("FPGA VI Reference In"=w42, "error in"=w41) -> ("error out"=w44:errorcluster)
  n179 = call <vilib>:"General Error Handler.vi"("error in (no error)"=w44) -> ()  [unwired: 10 in, 5 out]
